vi "calibrate trap data.vi"(4 "T2 cal":T1={"T2 alpha_x (nm/V)"=678.0121440160386, "T2 offset_x (mV)"=-14.421148336697543, "T2 kappa_x (pN/nm)"=0.2167951647771519} {"T2 kappa_x (pN/nm)" min=0.0 step=0.001 format="%#_2g"; "T2 offset_x (mV)" format="%#_2g"; "T2 alpha_x (nm/V)" step=10.0 format="%#_3g"}, 5 "T2":dbl[](array[numeric]), 6 "T1 cal":T2={"T1 alpha_x (nm/V)"=925.7792512885474, "T1 offset_x (mV)"=-22.37819181637641, "T1 kappa_x (pN/nm)"=0.15700163781152213} {"T1 kappa_x (pN/nm)" min=0.0 step=0.001 format="%#_2g"; "T1 offset_x (mV)" format="%#_2g"; "T1 alpha_x (nm/V)" step=10.0 format="%#_3g"}, 7 "T1":dbl[](array[numeric])) -> (0 "T2 force (pN)":dbl[](array[numeric]), 1 "T2 position (nm)":dbl[](array[numeric]), 2 "T1 force (pN)":dbl[](array[numeric]), 3 "T1 position (nm)":dbl[](array[numeric]))   [LabVIEW 2014]
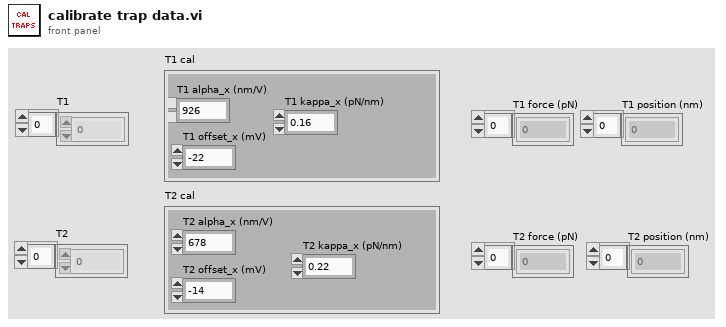
[diagram p1: front panel]
types:
  T1 = cluster{"T2 alpha_x (nm/V)":dbl, "T2 offset_x (mV)":dbl, "T2 kappa_x (pN/nm)":dbl}
  T2 = cluster{"T1 alpha_x (nm/V)":dbl, "T1 offset_x (mV)":dbl, "T1 kappa_x (pN/nm)":dbl}
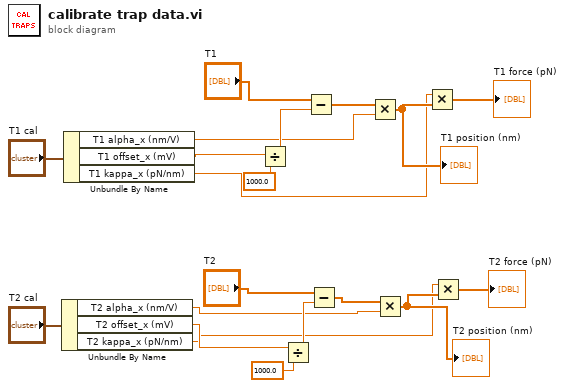
[diagram p0: block diagram]
diagram:
  n1 = Unbundle By Name("T2 cal") -> ("T2 alpha_x (nm/V)"=w3:dbl, "T2 offset_x (mV)"=w5:dbl, "T2 kappa_x (pN/nm)"=w1:dbl)
  n2 = Unbundle By Name("T1 cal") -> ("T1 alpha_x (nm/V)"=w4:dbl, "T1 offset_x (mV)"=w6:dbl, "T1 kappa_x (pN/nm)"=w2:dbl)
  n3 = Divide(x=w6, y=1000.0) -> (x/y=w18:dbl)
  n4 = Divide(x=w5, y=1000.0) -> (x/y=w17:dbl)
  n5 = Subtract(x="T1", y=w18) -> (x-y=w14:dbl[])
  n6 = Subtract(x="T2", y=w17) -> (x-y=w13:dbl[])
  n7 = Multiply(x=w14, y=w4) -> (x*y=w12:dbl[])
  "T1 position (nm)" <- w12
  n8 = Multiply(x=w13, y=w3) -> (x*y=w11:dbl[])
  "T2 position (nm)" <- w11
  n9 = Multiply(x=w2, y=w12) -> (x*y=→"T1 force (pN)":dbl[])
  n10 = Multiply(x=w1, y=w11) -> (x*y=→"T2 force (pN)":dbl[])
